vi "test.vi"() -> ()   [LabVIEW 2014]
uses:
  <vilib>/Platform/storage/Storage.llb/usiSequenceRepresentation.ctl
  <vilib>/Platform/storage/Storage.llb/usiOverwriteOptions.ctl
  <vilib>/Platform/storage/lvStorage.llb/_openStorageWithRootAutoDetect.vi
  <vilib>/Platform/storage/lvStorage.llb/xStorage/xStorageSupp/ErrorOut.vi
  <vilib>/Platform/storage/lvStorage.llb/_createOrGetExplicitChildObject.vi
  <vilib>/Platform/storage/lvStorage.llb/_createOrGetByNameExplicitChildObject.vi
  <vilib>/Platform/storage/lvStorage.llb/__saveFloat64Channel.vi
  <vilib>/Platform/storage/Storage.llb/__savePropString.vi
  <vilib>/Platform/storage/lvStorage.llb/_queryPropPoly.vi
  <vilib>/Platform/storage/lvStorage.llb/_queryPropString.vi
  <vilib>/Platform/storage/lvStorage.llb/_queryGenericObjects.vi
  <vilib>/Platform/storage/lvStorage.llb/_loadAllDdt.vi
  <vilib>/Platform/storage/lvStorage.llb/xStorage/Open Data Storage/Open Data Storage.xnode
  <vilib>/Platform/storage/lvStorage.llb/xStorage/Write Data/Write Data.xnode
  <vilib>/Platform/storage/lvStorage.llb/xStorage/Read Data/Read Data.xnode
panel:
  out "Array":dbl[](array[numeric])
  in  "file path":path
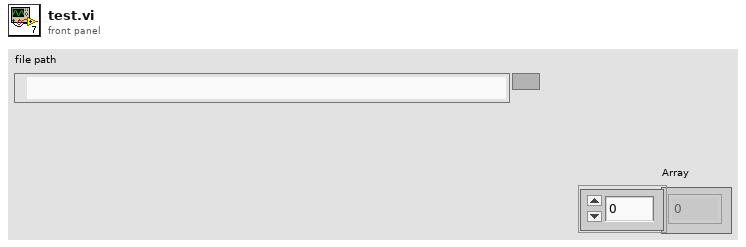
[diagram p1: front panel]
types:
  T1 = enum16{"open", "open or create", "create or replace", "create", "open (read only)"}
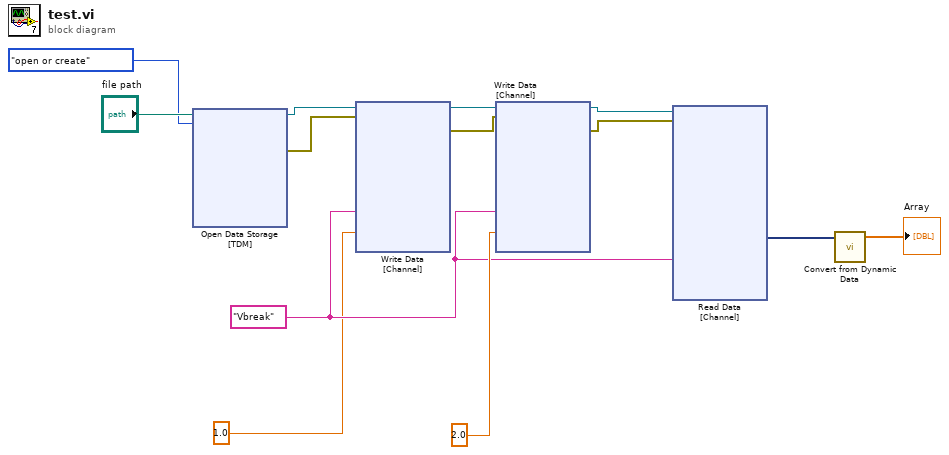
[diagram p0: block diagram]
diagram:
  w6 = "Vbreak" ("Name")
  n1 = xnode "Open Data Storage\n[TDM]"("file path"="file path", "function (open:0)"=T1."open or create") -> ("storage refnum (file)"=w13:refnum<k20>, "error out"=w12:errorcluster)  [unwired: 3 in, 1 out]
  n2 = xnode "Write Data\n[Channel]"("Name"=w6, "Signal"=1.0, "storage refnum (file)"=w13, "error in"=w12) -> ("storage refnum (file) out"=w11:refnum<k20>, "error out"=w10:errorcluster)  [unwired: 2 in, 1 out]
  n3 = xnode "Write Data\n[Channel]"("Name"=w6, "Signal"=2.0, "storage refnum (file)"=w11, "error in"=w10) -> ("storage refnum (file) out"=w8:refnum<k20>, "error out"=w7:errorcluster)  [unwired: 2 in, 1 out]
  n4 = xnode "Read Data\n[Channel]"("Name"=w6, "storage refnum (file)"=w8, "error in"=w7) -> ("Signal"=w3:dynamicdata)  [unwired: 3 in, 3 out]
  n5 = call "Convert from Dynamic Data"("Dynamic Data Type"=w3) -> ("Array"=→"Array":dbl[])  [unwired: 3 in]
